vi "FTW-Test-Timer.vi"() -> (0 "Test Result":errorcluster)   [LabVIEW 2015]
uses:
  src/error/FTW-ERR-ThrowError.vi
  src/error/FTW-ERR-CallChain.vi
  src/string/FTW-STR-ReplaceWhitespace.vi
  src/string/FTW-STR-Array-Delimit.vi
panel:
  out "Elapsed Time":dbl format="%.4psec"
  out "Waveform Graph":dbl[](graph)
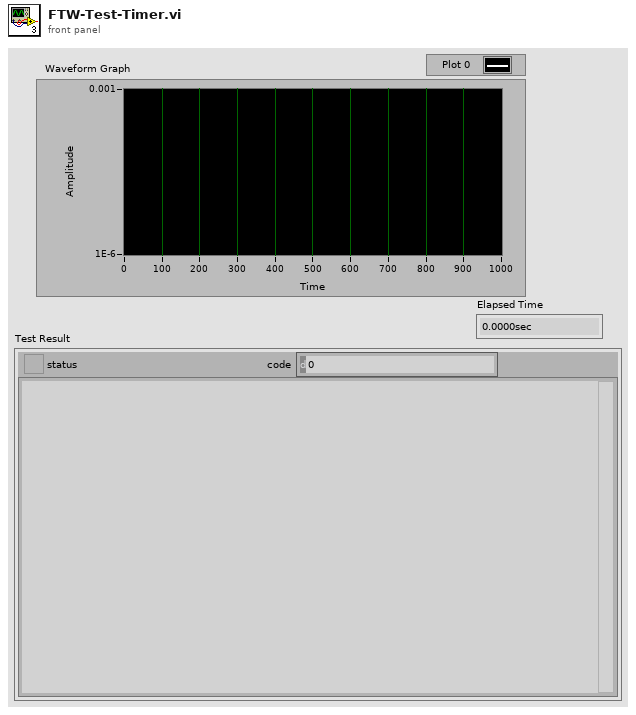
[diagram p1: front panel]
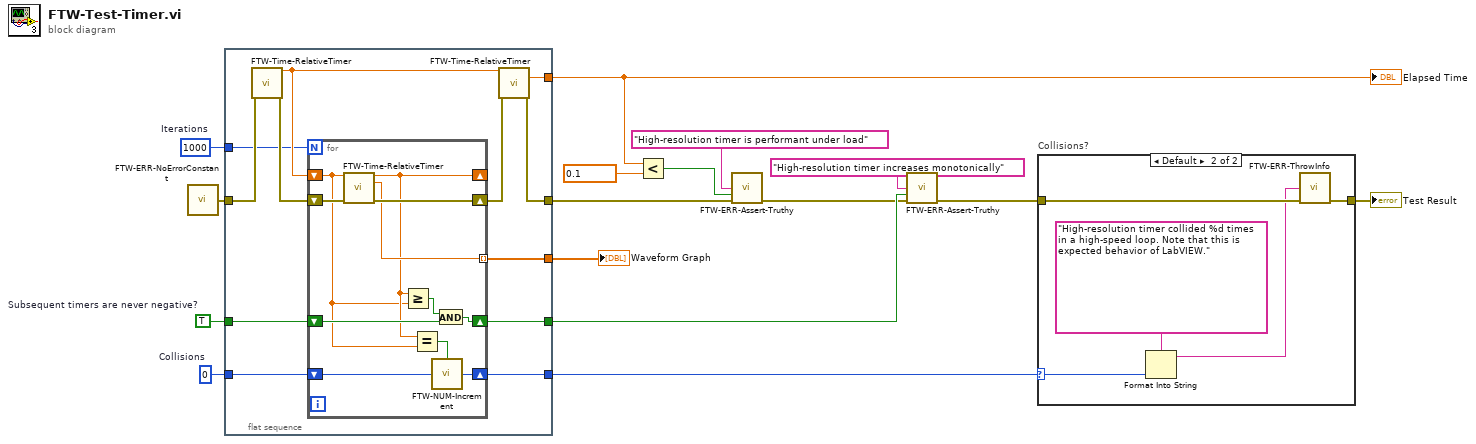
[diagram p0: block diagram]
diagram:
  w2 = 1000  # Iterations
  w3 = 0  # Collisions
  w1 = TRUE  # Subsequent timers are never negative?
  n1 = call "FTW-ERR-NoErrorConstant.vi"() -> ("no error"=w16:errorcluster)
  n2 = flat-sequence {
    tunnel: w16 -> [w28]
    tunnel: [w26] -> w15
    tunnel: [w23] -> w8
    tunnel: [w22] -> w14
    tunnel: [w21] -> w9
    tunnel: [w20] -> w4
    tunnel: w3 -> [w19]
    tunnel: w2 -> [w18]
    tunnel: w1 -> [w17]
    frame #0 {
      n3 = call "FTW-Time-RelativeTimer.vi"("error in"=w28) -> ("Current Timer Value"=w25:dbl, "error out"=w27:errorcluster)  [unwired: 12 in, 1 out]
      n4 = for {
        N: w18 -> [_]
        shift-right: [w33] -> _
        shift-left: w25 -> [w32]
        shift-right: [w38] -> w24
        shift-left: w27 -> [w39]
        tunnel: [w37] -> w26 mode=indexing
        shift-right: [w34] -> w21
        shift-left: w17 -> [w35]
        shift-right: [w29] -> w20
        shift-left: w19 -> [w30]
        n5 = call "FTW-Time-RelativeTimer.vi"("Previous Timer Value"=w32, "error in"=w39) -> ("Current Timer Value"=w33:dbl, "Elapsed Time"=w37:dbl, "error out"=w38:errorcluster)  [unwired: 11 in]
        n6 = Greater Or Equal?(x=w33, y=w32) -> (x >= y?=w36:bool)
        n7 = Equal?(x=w33, y=w32) -> (x = y?=w31:bool)
        n8 = call "FTW-NUM-Increment.vi"("Initial Value"=w30, "Increment?"=w31) -> ("Final Value"=w29:i32)
        n9 = And(x=w36, y=w35) -> (x .and. y?=w34:bool)
      }
      n10 = call "FTW-Time-RelativeTimer.vi"("Previous Timer Value"=w25, "error in"=w24) -> ("Elapsed Time"=w22:dbl, "error out"=w23:errorcluster)  [unwired: 11 in, 1 out]
    }
  }
  n11 = Less?(x=w14, y=0.1) -> (x < y?=w12:bool)
  n12 = call "FTW-ERR-Assert-Truthy.vi"("Assertion"="High-resolution timer is performant under load", "Assertion holds true?"=w12, "error in"=w8) -> ("error out"=w7:errorcluster)  [unwired: 12 in]
  n13 = call "FTW-ERR-Assert-Truthy.vi"("Assertion"="High-resolution timer increases monotonically", "Assertion holds true?"=w9, "error in"=w7) -> ("error out"=w6:errorcluster)  [unwired: 12 in]
  n14 = case "Collisions?" shown="Default" w4 {
    selector: w4 -> [_ w43]
    tunnel: w6 -> [w40 w45]
    tunnel: [w40 w44] -> w5
    frame 0 {
    }
    frame Default {
      n15 = Format Into String(format string="High-resolution timer collided %d times in a high-speed loop. Note that this is expected behavior of LabVIEW.", w43) -> (resulting string=w41:string)  [unwired: 2 in, 1 out]
      n16 = call "FTW-ERR-ThrowInfo.vi"("Informational Message"=w41, "error in"=w45) -> ("error out"=w44:errorcluster)  [unwired: 13 in]
    }
  }
  "Test Result" <- w5
  "Waveform Graph" <- w15
  "Elapsed Time" <- w14
